vi "PH_Cam_BaseClass.evt call SaveImage.vi"(0 "i ref in":refnum<vi>, 2 "Instance":string, 3 "Last/Next":bool, 4 "File refnum":refnum<file>, 5 "error in (no error)":errorcluster) -> (14 "i ref out":refnum<vi>, 19 "error out":errorcluster)   [LabVIEW 2014, in "PH_Cam_BaseClass.lvlib"]
doc: "This VI sends a simple call for SaveImg."
uses:
  CS_Core/CSSystem/CoreLib/CoreLib.string 2 byte array.vi
  CS_Core/CSSystem/CoreLib/CoreLib.short 2 byte array.vi
  PH_Cam_BaseClass.lvlib
  CS_Core/CSSystem/CoreLib/CoreLib.lvlib
  CS_Core/BaseProcess/BaseProcess.lvlib
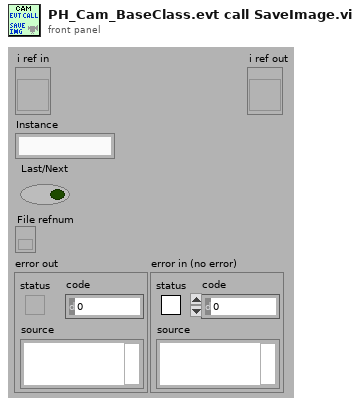
[diagram p1: front panel]
types:
  T1 = typedef "CoreDefs.rawDataType.ctl" = i8[]
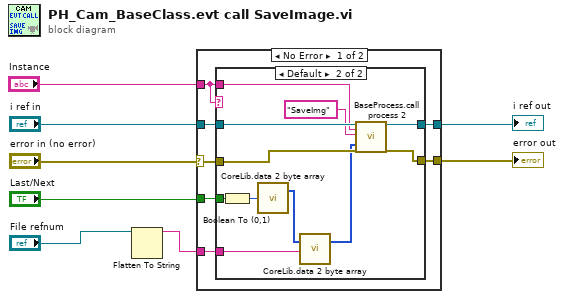
[diagram p0: block diagram]
diagram:
  n1 = Flatten To String(anything="File refnum") -> (data string=w3:string)  [unwired: 3 in, 2 out]
  n2 = case shown="No Error" "error in (no error)" {
    selector: "error in (no error)" -> [w11 w29]
    tunnel: [w15 w30] -> w2
    tunnel: [w14 w29] -> w1
    tunnel: "i ref in" -> [w13 w30]
    tunnel: "Instance" -> [w10 _]
    tunnel: "Last/Next" -> [w12 _]
    tunnel: w3 -> [w9 _]
    frame No Error {
      n3 = case shown="Default" w10 {
        tunnel: [w17 w28] -> w15
        tunnel: [w16 w27] -> w14
        tunnel: w13 -> [w17 w26]
        tunnel: w10 -> [_ w25]
        tunnel: w12 -> [_ w22]
        tunnel: w11 -> [w16 w21]
        tunnel: w9 -> [_ w18]
        frame "N/A" {
        }
        frame Default {
          n4 = Boolean To (0,1)(Boolean=w22) -> (0, 1=w23:i16)
          n5 = call-poly "CoreLib.data 2 byte array.vi"("i16"=w23) -> ("byteArray out"=w20:T1)  [unwired: 18 in]
          n6 = call-poly "CoreLib.data 2 byte array.vi"("byteArray"=w20, "string"=w18) -> ("byteArray out"=w19:T1)  [unwired: 17 in]
          n7 = call "BaseProcess.call process 2.vi"("i ref in"=w26, "Object"=w25, "Selector"="SaveImg", "Data"=w19, "error in (no error)"=w21) -> ("i ref out"=w28:refnum<vi>, "error out"=w27:errorcluster)  [unwired: 13 in]
        }
      }
    }
    frame Error {
    }
  }
  "error out" <- w1
  "i ref out" <- w2
